vi "Apply Theme To TitleBar-Splitter.vi"(8 "Error In":errorcluster, 9 "Override Root With (Empty)":string, 10 "Splitter Ref":refnum<vi>, 11 "ini Theme in":refnum<class "ini Theme.lvclass">) -> (0 "Error Out":errorcluster, 3 "ini Theme out":refnum<class "ini Theme.lvclass">)   [LabVIEW 2021, in "Appearance Actor.lvlib" / "ini Theme.lvclass"]
uses:
  ini Theme.lvclass
  Generic Theme/API/Typedefs/Theme Entry--enum.ctl
  ini Theme.lvclass/ini Theme.ctl
  fa3b262b-9dee-4a2a-a40e-e8b24c2842d1.vi
  e580e7d3-37e0-4797-b7d4-6ea3cff1905c.vi
  0ddc5fb1-c68a-4eb1-8b3f-3a92131e0179.vi
  d2827a1e-72b6-49ff-b445-8daa62495d43.vi
  <vilib>/Utility/config.llb/Read Key (U32).vi
  <vilib>/Utility/config.llb/NI_LVConfig.lvlib
  Generic Theme/Generic Theme.lvclass
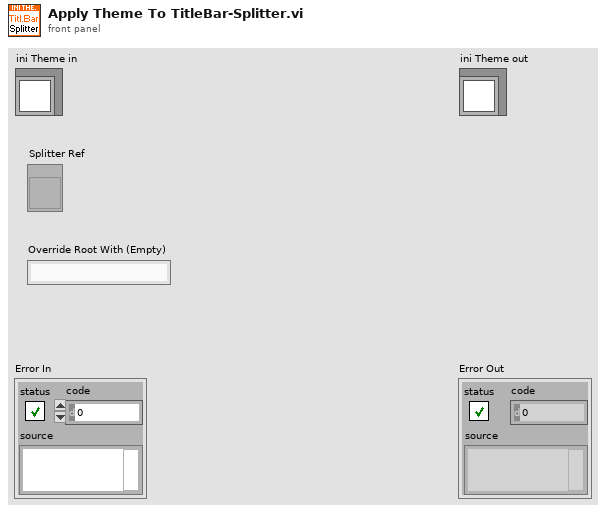
[diagram p1: front panel]
types:
  T1 = typedef "Appearance Actor.lvlib/Generic Theme.lvclass/Theme Entry--enum.ctl" = enum16{"None", "TitleBar.Pane.Color", "TitleBar.Splitter.FillColor", "TitleBar.Splitter.OutlineColor", "TitleBar.Title.Font.Color", "TitleBar.Title.Font.Family", "TitleBar.Title.Font.Size", "TitleBar.Title.Font.Style"}
  T2 = typedef "NI_LVConfig.lvlib/Config Data RefNum.ctl" = refnum<k1>
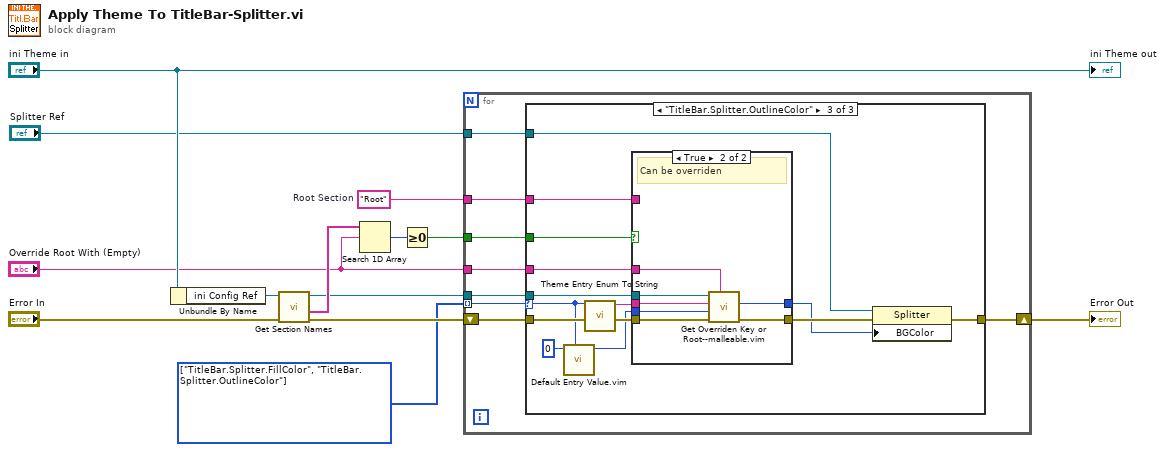
[diagram p0: block diagram]
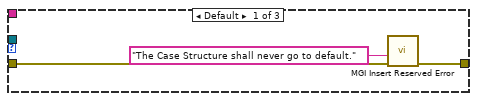
[diagram p2: hidden frame]
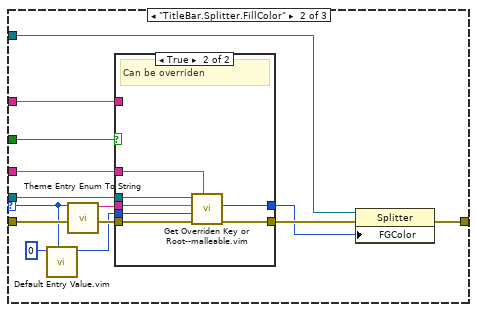
[diagram p3: hidden frame]
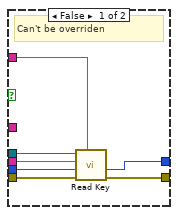
[diagram p4: hidden frame]
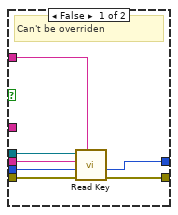
[diagram p5: hidden frame]
diagram:
  w2 = T1[] [enum."TitleBar.Splitter.FillColor", enum."TitleBar.Splitter.OutlineColor"] items=["None", "TitleBar.Pane.Color", "TitleBar.Splitter.FillColor", "TitleBar.Splitter.OutlineColor", "TitleBar.Title.Font.Color", "TitleBar.Title.Font.Family", "TitleBar.Title.Font.Size", "TitleBar.Title.Font.Style"] ("Array")
  w3 = "Root"  # Root Section
  n1 = Unbundle By Name("ini Theme in") -> ("ini Config Ref"=w13:T2)
  n2 = call <vilib>:"Get Section Names.vi"("error in (no error)"="Error In", "refnum"=w13) -> ("error out"=w10:errorcluster, "section names"=w12:string[], "refnum out"=w4:T2)  [unwired: 7 in]
  n3 = Search 1D Array(1D array=w12, element="Override Root With (Empty)") -> (index of element=w11:i32)  [unwired: 1 in]
  n4 = Greater Or Equal To 0?(x=w11) -> (x >= 0?=w5:bool)
  n5 = for {
    shift-right: [w15] -> w8
    shift-left: w10 -> [w21]
    tunnel: "Override Root With (Empty)" -> [w20]
    tunnel: w5 -> [w19]
    tunnel: w4 -> [w18]
    tunnel: w3 -> [w17]
    tunnel: w2 -> [w16] mode=indexing
    tunnel: "Splitter Ref" -> [w14]
    n6 = case shown="\"TitleBar.Splitter.OutlineColor\"" w16 {
      selector: w16 -> [_ w25 w52]
      tunnel: w21 -> [w23 w37 w64]
      tunnel: w20 -> [_ w35 w62]
      tunnel: w19 -> [_ w34 w61]
      tunnel: w18 -> [_ w33 w60]
      tunnel: w17 -> [_ w32 w59]
      tunnel: [w22 w31 w58] -> w15
      tunnel: w14 -> [_ w30 w57]
      frame Default {
        n7 = call <userlib>:"MGI Insert Reserved Error.vi"("Error In"=w23, "Error Description"="The Case Structure shall never go to default.") -> ("Error Out"=w22:errorcluster)  [unwired: 9 in]
      }
      frame "TitleBar.Splitter.FillColor" {
        n8 = call "Default Entry Value.vim"("Root Theme Entry"=w25, "Data Type"=u32 0) -> ("Default Value"=w27:u32)  [unwired: 9 in]
        n9 = call "Theme Entry Enum To String.vi"("Root Theme Entry"=w25) -> ("Root Theme Entry String"=w28:string)  [unwired: 10 in]
        n10 = case shown="True" w34 {
          tunnel: w37 -> [w44 w51]
          tunnel: [w43 w50] -> w36
          tunnel: w35 -> [_ w49]
          tunnel: w33 -> [w41 w48]
          tunnel: w32 -> [w42 _]
          tunnel: w28 -> [w40 w47]
          tunnel: w27 -> [w38 w46]
          tunnel: [w39 w45] -> w29
          frame False {
            # "Can't be overriden"
            n11 = call-poly <vilib>:"Read Key.vi"("section"=w42, "error in (no error)"=w44, "default value"=w38, "key"=w40, "refnum"=w41) -> ("error out"=w43:errorcluster, "value"=w39:u32)  [unwired: 3 in, 2 out]
          }
          frame True {
            # "Can be overriden"
            n12 = call "Get Overriden Key or Root--malleable.vim"("Override Root With"=w49, "Error In"=w51, "Default"=w46, "Key"=w47, "ini Ref In"=w48) -> ("Error Out"=w50:errorcluster, "Value"=w45:u32)  [unwired: 4 in, 1 out]
          }
        }
        n13 = property class="Splitter"(reference=w30, error in=w36, "FGColor"=w29) -> (error out=w31:errorcluster)  [unwired: 1 out]
      }
      frame "TitleBar.Splitter.OutlineColor" {
        n14 = call "Default Entry Value.vim"("Root Theme Entry"=w52, "Data Type"=u32 0) -> ("Default Value"=w54:u32)  [unwired: 9 in]
        n15 = call "Theme Entry Enum To String.vi"("Root Theme Entry"=w52) -> ("Root Theme Entry String"=w55:string)  [unwired: 10 in]
        n16 = case shown="True" w61 {
          tunnel: w64 -> [w71 w78]
          tunnel: [w70 w77] -> w63
          tunnel: w62 -> [_ w76]
          tunnel: w60 -> [w68 w75]
          tunnel: w59 -> [w69 _]
          tunnel: w55 -> [w67 w74]
          tunnel: w54 -> [w65 w73]
          tunnel: [w66 w72] -> w56
          frame False {
            # "Can't be overriden"
            n17 = call-poly <vilib>:"Read Key.vi"("section"=w69, "error in (no error)"=w71, "default value"=w65, "key"=w67, "refnum"=w68) -> ("error out"=w70:errorcluster, "value"=w66:u32)  [unwired: 3 in, 2 out]
          }
          frame True {
            # "Can be overriden"
            n18 = call "Get Overriden Key or Root--malleable.vim"("Override Root With"=w76, "Error In"=w78, "Default"=w73, "Key"=w74, "ini Ref In"=w75) -> ("Error Out"=w77:errorcluster, "Value"=w72:u32)  [unwired: 4 in, 1 out]
          }
        }
        n19 = property class="Splitter"(reference=w57, error in=w63, "BGColor"=w56) -> (error out=w58:errorcluster)  [unwired: 1 out]
      }
    }
  }
  "Error Out" <- w8
  "ini Theme out" <- "ini Theme in"
